vi "Calc U from Re.vi"(4 "Wire diameter (m)":dbl=5e-06, 6 "T0 (°C)":dbl=20.0, 8 "alpha0 (/°C)":dbl=0.0036, 9 "Overheat ratio (Rw / R0)":dbl=1.7, 10 "Ta (°C)":dbl=25.0, 11 "Re":dbl=1.0) -> (3 "U (m/s)":dbl=5.134553282523611)   [LabVIEW 2022 SP3]
doc: "Calculate U from Re (taking into account Ta).\nPN 05-NOV-23."
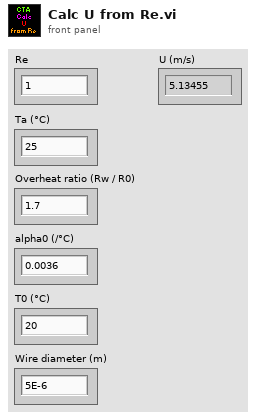
[diagram p1: front panel]
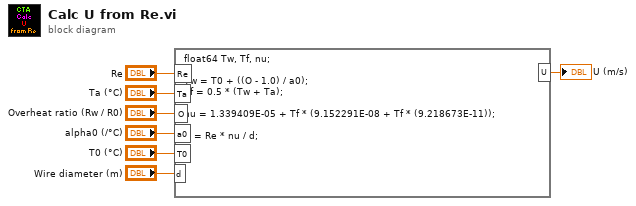
[diagram p0: block diagram]
diagram:
  n1 = formula code="float64 Tw, Tf, nu;\n\nTw = T0 + ((O - 1.0) / a0);\nTf = 0.5 * (Tw + Ta);\n\nnu = 1.339409E-05 + Tf * (9.152291E-08 + Tf * (9.218673E-11));\n\nU = Re * nu / d;"("Re"="Re", "Ta"="Ta (°C)", "O"="Overheat ratio (Rw / R0)", "a0"="alpha0 (/°C)", "T0"="T0 (°C)", "d"="Wire diameter (m)") -> ("U"=→"U (m/s)":dbl)
